vi "Call Measure.vi"(0 "Measurement Client Wrapper in":refnum<class "Measurement Client Wrapper.lvclass">, 5 "Config Data":T2(array[cluster]), 7 "Expected Output Format":T2(array[cluster]), 9 "ConfigurationParametersMessagetype":string, 11 "error in (no error)":errorcluster) -> (4 "Measurement Client Wrapper out":refnum<class "Measurement Client Wrapper.lvclass">, 6 "Output Data":T2(array[cluster]), 15 "error out":errorcluster)   [LabVIEW 2020, in "Measurement Client Wrapper.lvclass"]
uses:
  Measurement Client Wrapper.lvclass
  Typedefs/Measurement DataType.ctl
  Measurement Client Wrapper.lvclass/Measurement Client Wrapper.ctl
  <vilib>/gRPC/LabVIEW gRPC Library/Server API/typeDefs/Message Element Type.ctl
  02400f1b-8973-4b95-8741-fbceca04c3fe.vi
  5b726686-77e5-40ef-be8d-2074d1d57e99.vi
  95b28ee5-f8e2-4b34-8d76-37da75901063.vi
  00fa3f71-b6c4-4477-9b91-f6e537aa3dd8.vi
  5907dd95-356c-493c-a4fb-246df12ff7d4.vi
  c2266674-1d71-4ea2-b566-157aa4afc0f2.vi
  1a1b2748-f9f2-4ce1-9d96-6eb652a988f1.vi
  d543a457-6964-494b-8b0b-6a35ff49fad2.vi
  99282071-cc29-4e12-a9c1-055a10bff9dc.vi
  d266cb79-5d95-441f-85b0-bd6ef5cfb0df.vi
  03ab3711-fcfd-4277-a820-7570fda2cb30.vi
  0c734c18-9f5b-4fb1-9d32-7552b2f84713.vi
  e636cc20-c55c-4ee7-9f06-d3ba27ad9f12.vi
  7d8d1cdd-67f0-488f-acda-45a393ef5429.vi
  dec23bc4-0ee6-41f8-bde8-6d2a7e7bdfda.vi
  0367a431-a951-4815-abe7-6dcef05fe4c8.vi
  10f836c9-6199-4ce1-a626-5162e79beb86.vi
  96ee5240-0b84-4974-8ad0-9b306673ed4a.vi
  d29134f8-404b-4b6f-a3af-5734ff761ebd.vi
  181fb914-151b-4e06-975b-9dc9e5afafa5.vi
  588d01ac-b7df-4f6b-8274-d762d09c065e.vi
  c5a5b341-584b-41e8-87a1-35fc57d4ddfd.vi
  f3bca736-9bdf-40e5-ab0d-7db104ab277d.vi
  6802ca25-6fd7-49a0-8882-e0466137b412.vi
  c7c6e655-8529-4469-afec-6f432153ed64.vi
  520864e9-ee10-48de-be12-7897d471816d.vi
  46e9815d-b5c5-41d7-ada4-ba252c25d075.vi
  bc126205-1da4-432e-a22b-db4c055c1324.vi
  e14ad0fc-2d1f-4c15-8e45-af447a0faebc.vi
  407f5415-5085-4ddd-a591-6d04ba5119ca.vi
  af61a386-2c35-4d4b-91aa-3cbffd5e8033.vi
  97c6c522-6e58-44d8-a6ef-9522c331f38e.vi
  <vilib>/gRPC/LabVIEW gRPC Library/Server API/Server/Get Server DLL Path.vi
  Measurement_lv_client/Measurement_lv_client Class/Measurement_lv_client.lvclass
  <vilib>/gRPC/LabVIEW gRPC Library/gprc-lvsupport-release.lvlib
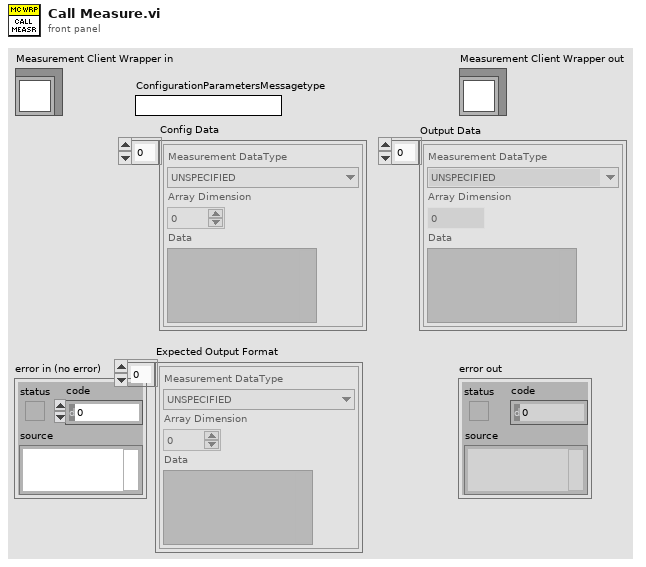
[diagram p1: front panel]
types:
  T1 = typedef "Measurement Client Wrapper.lvclass/Measurement DataType.ctl" = enum16{"UNSPECIFIED", "BOOL", "DOUBLE", "FLOAT", "INT32", "INT64", "STRING", "UINT32", "UINT64"}
  T2 = cluster{"Measurement DataType":T1, "Array Dimension":i32, "Data":variant}[]
  T3 = typedef "gprc-lvsupport-release.lvlib/Message Element Type.ctl" = enum32{"Int32Value", "FloatValue", "DoubleValue", "BoolValue", "StringValue", "MessageValue", "Int64Value", "UInt32Value", "UInt64Value", "EnumValue", "Bytes", "Fixed64", "Fixed32", "SFixed64", "SFixed32", "SInt64", "SInt32"}
  T4 = typedef "gprc-lvsupport-release.lvlib/grpcId.ctl" = u64
  T5 = typedef "Measurement_lv_client.lvlib/Measurement_lv_client.lvclass/Measurement_v1_MeasureResponse_Data.ctl" = cluster{"outputs":T6, "Error":T7}
  T6 = typedef "Measurement_lv_client.lvlib/Measurement_lv_client.lvclass/google_protobuf_Any_Data.ctl" = cluster{"type_url":string, "value":u8[]}
  T7 = typedef "Measurement_lv_client.lvlib/Measurement_lv_client.lvclass/Measurement_v1_ErrorInformation_Data.ctl" = cluster{"iserror":bool, "errorcode":i32, "errordetails":string}
  T8 = cluster{"Measurement DataType":T1, "Array Dimension":i32, "Data":variant}
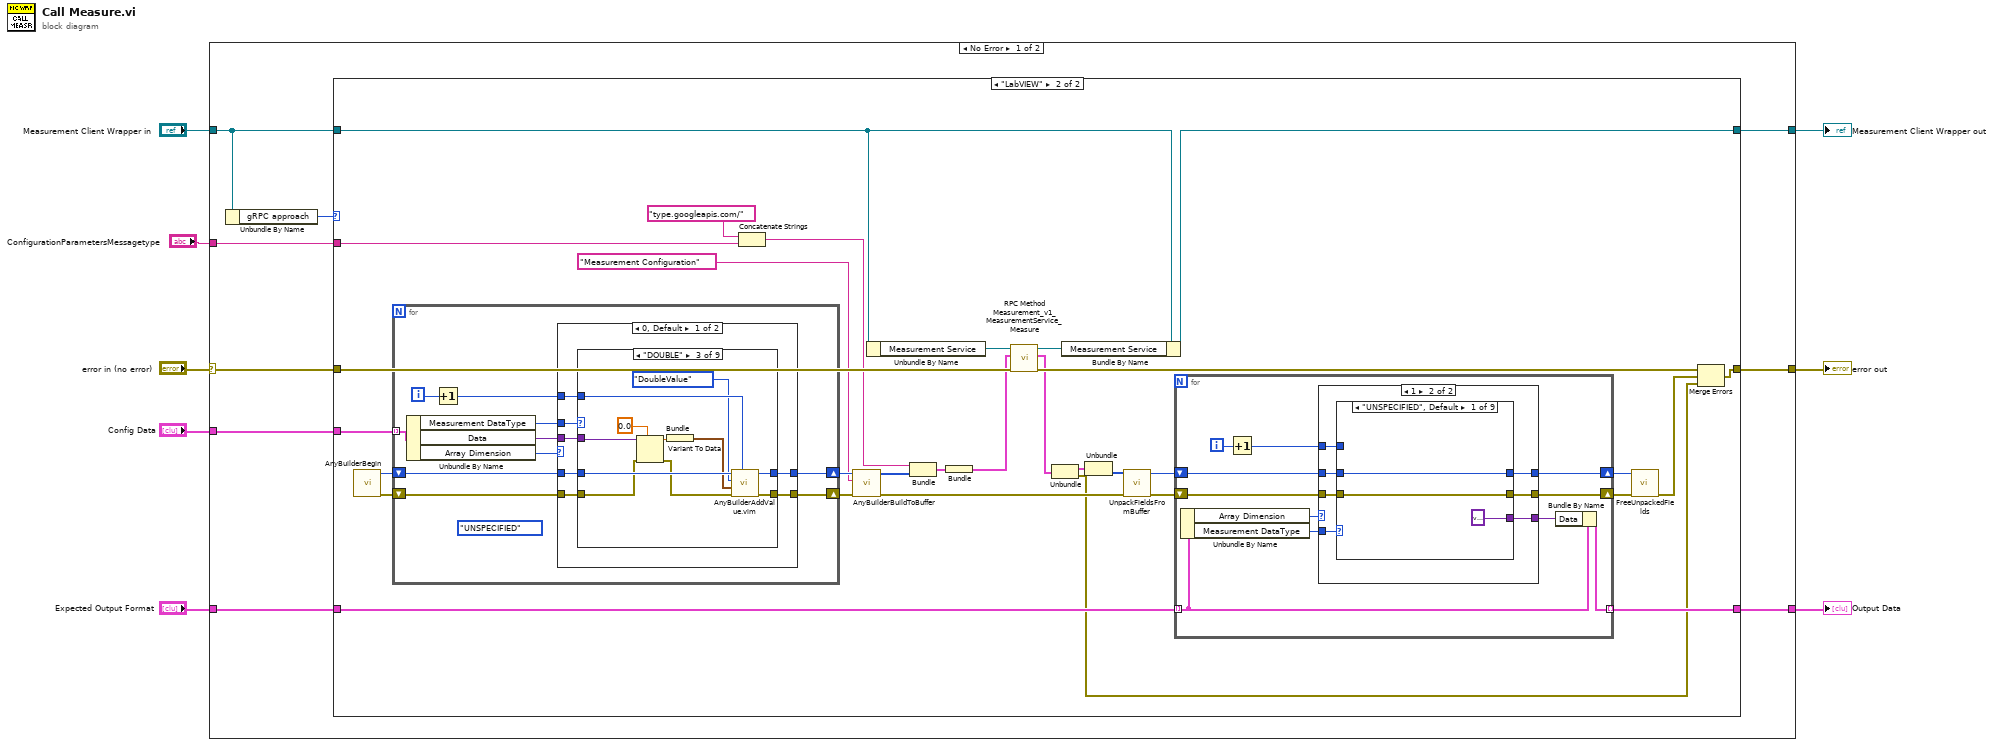
[diagram p0: block diagram]
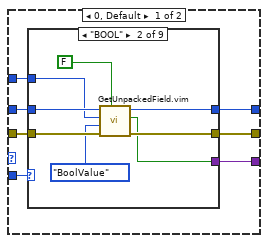
[diagram p3: hidden frame]
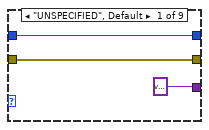
[diagram p4: hidden frame]
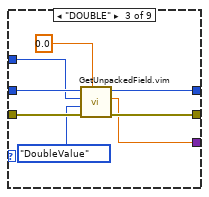
[diagram p5: hidden frame]
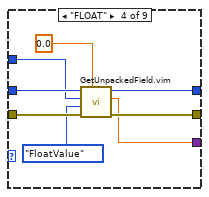
[diagram p6: hidden frame]
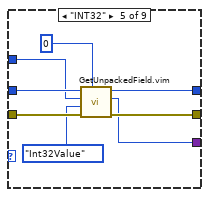
[diagram p7: hidden frame]
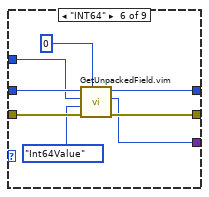
[diagram p8: hidden frame]
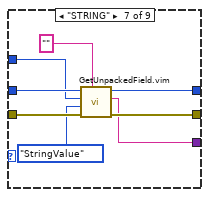
[diagram p9: hidden frame]
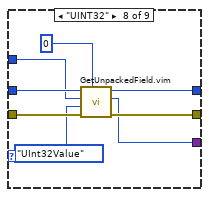
[diagram p10: hidden frame]
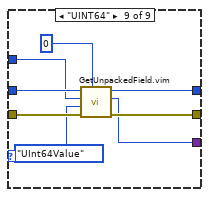
[diagram p11: hidden frame]
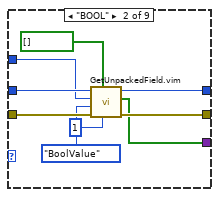
[diagram p12: hidden frame]
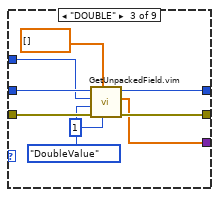
[diagram p13: hidden frame]
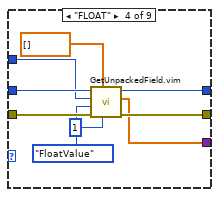
[diagram p14: hidden frame]
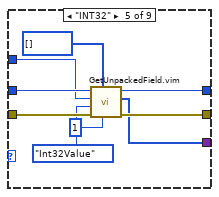
[diagram p15: hidden frame]
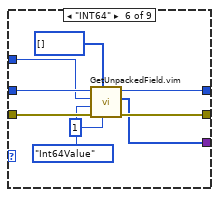
[diagram p16: hidden frame]
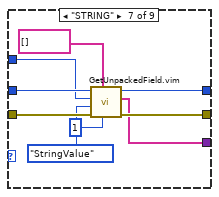
[diagram p17: hidden frame]
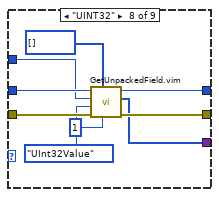
[diagram p18: hidden frame]
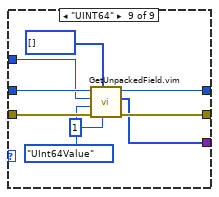
[diagram p19: hidden frame]
diagram:
  n1 = case shown="No Error" "error in (no error)" {
    selector: "error in (no error)" -> [w17 w432]
    tunnel: [w16 w432] -> w7
    tunnel: [w15 w431] -> w5
    tunnel: "Measurement Client Wrapper in" -> [w14 w431]
    tunnel: "Config Data" -> [w12 _]
    tunnel: "Expected Output Format" -> [w11 _]
    tunnel: [w10 _] -> w2
    tunnel: "ConfigurationParametersMessagetype" -> [w9 _]
    frame No Error {
      n2 = Unbundle By Name(w14) -> ("gRPC approach"=w13:enum16{".NET", "LabVIEW"})
      n3 = case shown="\"LabVIEW\"" w13 {
        tunnel: w17 -> [w20 w50]
        tunnel: [w20 w37] -> w16
        tunnel: [w19 w47] -> w15
        tunnel: w14 -> [w19 w48]
        tunnel: w12 -> [_ w45]
        tunnel: w11 -> [w18 w32]
        tunnel: [w18 w29] -> w10
        tunnel: w9 -> [_ w21]
        frame ".NET", Default {
        }
        frame "LabVIEW" {
          n4 = call <vilib>:"AnyBuilderBegin.vi"() -> ("error out"=w44:errorcluster, "Builder Ref Out"=w43:T4)  [unwired: 9 in]
          n5 = for {
            tunnel: w45 -> [w228] mode=indexing
            shift-right: [w222] -> w41
            shift-left: w44 -> [w221]
            shift-right: [w223] -> w42
            shift-left: w43 -> [w224]
            i -> [w227]
            (unwired) Measurement_DataType."UNSPECIFIED" ("Measurement DataType")
            n6 = Unbundle By Name(w228) -> ("Measurement DataType"=w226:T1, "Data"=w225:variant, "Array Dimension"=w219:i32)
            n7 = Increment(x=w227) -> (x+1=w220:i32)
            n8 = case shown="0, Default" w219 {
              tunnel: w226 -> [w235 w332]
              tunnel: w225 -> [w234 w331]
              tunnel: w224 -> [w233 w330]
              tunnel: [w232 w329] -> w223
              tunnel: [w231 w328] -> w222
              tunnel: w221 -> [w230 w327]
              tunnel: w220 -> [w229 w326]
              frame 0, Default {
                n9 = case shown="\"DOUBLE\"" w235 {
                  tunnel: w234 -> [_ w243 w254 w265 w276 w287 w298 w309 w320]
                  tunnel: w233 -> [w237 w248 w259 w270 w281 w292 w303 w314 w325]
                  tunnel: [w237 w247 w258 w269 w280 w291 w302 w313 w324] -> w232
                  tunnel: [w236 w246 w257 w268 w279 w290 w301 w312 w323] -> w231
                  tunnel: w230 -> [w236 w241 w253 w264 w275 w286 w297 w308 w319]
                  tunnel: w229 -> [_ w245 w256 w267 w278 w289 w300 w311 w322]
                  frame "UNSPECIFIED", Default {
                  }
                  frame "BOOL" {
                    n10 = Variant To Data(error in=w241, type=TRUE, Variant=w243) -> (data=w239:bool, error out=w240:errorcluster)
                    n11 = Bundle(w239) -> (w238:cluster{bool})  [unwired: 1 in]
                    n12 = call "AnyBuilderAddValue.vim"("protobufId"=w245, "error in (no error)"=w240, "Value"=w238, "MessageElementType"=Message_Element_Type."BoolValue", "gRPCid in"=w248) -> ("error out"=w246:errorcluster, "gRPCid"=w247:u64)  [unwired: 5 in]
                  }
                  frame "DOUBLE" {
                    n13 = Variant To Data(error in=w253, type=0.0, Variant=w254) -> (data=w249:dbl, error out=w252:errorcluster)
                    n14 = Bundle(w249) -> (w251:cluster{dbl})  [unwired: 1 in]
                    n15 = call "AnyBuilderAddValue.vim"("protobufId"=w256, "error in (no error)"=w252, "Value"=w251, "MessageElementType"=Message_Element_Type."DoubleValue", "gRPCid in"=w259) -> ("error out"=w257:errorcluster, "gRPCid"=w258:u64)  [unwired: 5 in]
                  }
                  frame "FLOAT" {
                    n16 = Variant To Data(error in=w264, type=sgl 0.0, Variant=w265) -> (data=w261:sgl, error out=w263:errorcluster)
                    n17 = Bundle(w261) -> (w260:cluster{sgl})  [unwired: 1 in]
                    n18 = call "AnyBuilderAddValue.vim"("protobufId"=w267, "error in (no error)"=w263, "Value"=w260, "MessageElementType"=Message_Element_Type."FloatValue", "gRPCid in"=w270) -> ("error out"=w268:errorcluster, "gRPCid"=w269:u64)  [unwired: 5 in]
                  }
                  frame "INT32" {
                    n19 = Variant To Data(error in=w275, type=0, Variant=w276) -> (data=w272:i32, error out=w274:errorcluster)
                    n20 = Bundle(w272) -> (w271:cluster{i32})  [unwired: 1 in]
                    n21 = call "AnyBuilderAddValue.vim"("protobufId"=w278, "error in (no error)"=w274, "Value"=w271, "MessageElementType"=Message_Element_Type."Int32Value", "gRPCid in"=w281) -> ("error out"=w279:errorcluster, "gRPCid"=w280:u64)  [unwired: 5 in]
                  }
                  frame "INT64" {
                    n22 = Variant To Data(error in=w286, type=i64 0, Variant=w287) -> (data=w283:i64, error out=w285:errorcluster)
                    n23 = Bundle(w283) -> (w282:cluster{i64})  [unwired: 1 in]
                    n24 = call "AnyBuilderAddValue.vim"("protobufId"=w289, "error in (no error)"=w285, "Value"=w282, "MessageElementType"=Message_Element_Type."Int64Value", "gRPCid in"=w292) -> ("error out"=w290:errorcluster, "gRPCid"=w291:u64)  [unwired: 5 in]
                  }
                  frame "STRING" {
                    n25 = Variant To Data(error in=w297, type="", Variant=w298) -> (data=w294:string, error out=w296:errorcluster)
                    n26 = Bundle(w294) -> (w293:cluster{string})  [unwired: 1 in]
                    n27 = call "AnyBuilderAddValue.vim"("protobufId"=w300, "error in (no error)"=w296, "Value"=w293, "MessageElementType"=Message_Element_Type."StringValue", "gRPCid in"=w303) -> ("error out"=w301:errorcluster, "gRPCid"=w302:u64)  [unwired: 5 in]
                  }
                  frame "UINT32" {
                    n28 = Variant To Data(error in=w308, type=u32 0, Variant=w309) -> (data=w305:u32, error out=w307:errorcluster)
                    n29 = Bundle(w305) -> (w304:cluster{u32})  [unwired: 1 in]
                    n30 = call "AnyBuilderAddValue.vim"("protobufId"=w311, "error in (no error)"=w307, "Value"=w304, "MessageElementType"=Message_Element_Type."UInt32Value", "gRPCid in"=w314) -> ("error out"=w312:errorcluster, "gRPCid"=w313:u64)  [unwired: 5 in]
                  }
                  frame "UINT64" {
                    n31 = Variant To Data(error in=w319, type=u64 0, Variant=w320) -> (data=w316:u64, error out=w318:errorcluster)
                    n32 = Bundle(w316) -> (w315:cluster{u64})  [unwired: 1 in]
                    n33 = call "AnyBuilderAddValue.vim"("protobufId"=w322, "error in (no error)"=w318, "Value"=w315, "MessageElementType"=Message_Element_Type."UInt64Value", "gRPCid in"=w325) -> ("error out"=w323:errorcluster, "gRPCid"=w324:u64)  [unwired: 5 in]
                  }
                }
              }
              frame 1 {
                n34 = case shown="\"BOOL\"" w332 {
                  tunnel: w331 -> [_ w341 w353 w365 w377 w389 w401 w413 w425]
                  tunnel: w330 -> [w334 w346 w358 w370 w382 w394 w406 w418 w430]
                  tunnel: [w334 w345 w357 w369 w381 w393 w405 w417 w429] -> w329
                  tunnel: [w333 w344 w356 w368 w380 w392 w404 w416 w428] -> w328
                  tunnel: w327 -> [w333 w340 w352 w364 w376 w388 w400 w412 w424]
                  tunnel: w326 -> [_ w343 w355 w367 w379 w391 w403 w415 w427]
                  frame "UNSPECIFIED", Default {
                  }
                  frame "BOOL" {
                    n35 = Variant To Data(error in=w340, type=bool[] [], Variant=w341) -> (data=w338:bool[], error out=w339:errorcluster)
                    n36 = Bundle(w338) -> (w337:cluster{bool[]})  [unwired: 1 in]
                    n37 = call "AnyBuilderAddValue.vim"("isRepeated"=1, "protobufId"=w343, "error in (no error)"=w339, "Value"=w337, "MessageElementType"=Message_Element_Type."BoolValue", "gRPCid in"=w346) -> ("error out"=w344:errorcluster, "gRPCid"=w345:u64)  [unwired: 4 in]
                  }
                  frame "DOUBLE" {
                    n38 = Variant To Data(error in=w352, type=dbl[] [], Variant=w353) -> (data=w349:dbl[], error out=w351:errorcluster)
                    n39 = Bundle(w349) -> (w350:cluster{dbl[]})  [unwired: 1 in]
                    n40 = call "AnyBuilderAddValue.vim"("isRepeated"=1, "protobufId"=w355, "error in (no error)"=w351, "Value"=w350, "MessageElementType"=Message_Element_Type."DoubleValue", "gRPCid in"=w358) -> ("error out"=w356:errorcluster, "gRPCid"=w357:u64)  [unwired: 4 in]
                  }
                  frame "FLOAT" {
                    n41 = Variant To Data(error in=w364, type=sgl[] [], Variant=w365) -> (data=w362:sgl[], error out=w363:errorcluster)
                    n42 = Bundle(w362) -> (w361:cluster{sgl[]})  [unwired: 1 in]
                    n43 = call "AnyBuilderAddValue.vim"("isRepeated"=1, "protobufId"=w367, "error in (no error)"=w363, "Value"=w361, "MessageElementType"=Message_Element_Type."FloatValue", "gRPCid in"=w370) -> ("error out"=w368:errorcluster, "gRPCid"=w369:u64)  [unwired: 4 in]
                  }
                  frame "INT32" {
                    n44 = Variant To Data(error in=w376, type=i32[] [], Variant=w377) -> (data=w374:i32[], error out=w375:errorcluster)
                    n45 = Bundle(w374) -> (w373:cluster{i32[]})  [unwired: 1 in]
                    n46 = call "AnyBuilderAddValue.vim"("isRepeated"=1, "protobufId"=w379, "error in (no error)"=w375, "Value"=w373, "MessageElementType"=Message_Element_Type."Int32Value", "gRPCid in"=w382) -> ("error out"=w380:errorcluster, "gRPCid"=w381:u64)  [unwired: 4 in]
                  }
                  frame "INT64" {
                    n47 = Variant To Data(error in=w388, type=i64[] [], Variant=w389) -> (data=w386:i64[], error out=w387:errorcluster)
                    n48 = Bundle(w386) -> (w385:cluster{i64[]})  [unwired: 1 in]
                    n49 = call "AnyBuilderAddValue.vim"("isRepeated"=1, "protobufId"=w391, "error in (no error)"=w387, "Value"=w385, "MessageElementType"=Message_Element_Type."Int64Value", "gRPCid in"=w394) -> ("error out"=w392:errorcluster, "gRPCid"=w393:u64)  [unwired: 4 in]
                  }
                  frame "STRING" {
                    n50 = Variant To Data(error in=w400, type=string[] [], Variant=w401) -> (data=w398:string[], error out=w399:errorcluster)
                    n51 = Bundle(w398) -> (w397:cluster{string[]})  [unwired: 1 in]
                    n52 = call "AnyBuilderAddValue.vim"("isRepeated"=1, "protobufId"=w403, "error in (no error)"=w399, "Value"=w397, "MessageElementType"=Message_Element_Type."StringValue", "gRPCid in"=w406) -> ("error out"=w404:errorcluster, "gRPCid"=w405:u64)  [unwired: 4 in]
                  }
                  frame "UINT32" {
                    n53 = Variant To Data(error in=w412, type=u32[] [], Variant=w413) -> (data=w410:u32[], error out=w411:errorcluster)
                    n54 = Bundle(w410) -> (w409:cluster{u32[]})  [unwired: 1 in]
                    n55 = call "AnyBuilderAddValue.vim"("isRepeated"=1, "protobufId"=w415, "error in (no error)"=w411, "Value"=w409, "MessageElementType"=Message_Element_Type."UInt32Value", "gRPCid in"=w418) -> ("error out"=w416:errorcluster, "gRPCid"=w417:u64)  [unwired: 4 in]
                  }
                  frame "UINT64" {
                    n56 = Variant To Data(error in=w424, type=u64[] [], Variant=w425) -> (data=w422:u64[], error out=w423:errorcluster)
                    n57 = Bundle(w422) -> (w421:cluster{u64[]})  [unwired: 1 in]
                    n58 = call "AnyBuilderAddValue.vim"("isRepeated"=1, "protobufId"=w427, "error in (no error)"=w423, "Value"=w421, "MessageElementType"=Message_Element_Type."UInt64Value", "gRPCid in"=w430) -> ("error out"=w428:errorcluster, "gRPCid"=w429:u64)  [unwired: 4 in]
                  }
                }
              }
            }
          }
          n59 = Concatenate Strings("type.googleapis.com/", w21) -> (w22:string)
          n60 = call <vilib>:"AnyBuilderBuildToBuffer.vi"("error in (no error)"=w41, "Message Type"="Measurement Configuration", "Builder Ref"=w42) -> ("error out"=w33:errorcluster, "Buffer"=w40:u8[])  [unwired: 7 in]
          n61 = Unbundle By Name(w48) -> ("Measurement Service"=w51:refnum<class "Measurement_lv_client.lvclass">)
          n62 = Bundle(w22, "Buffer"=w40) -> (w39:cluster{string, "Buffer":u8[]})  [unwired: 1 in]
          n63 = Bundle(w39) -> (w38:cluster{cluster{string, "Buffer":u8[]}})  [unwired: 1 in]
          n64 = call "RPC Method Measurement_v1_MeasurementService_Measure.vi"("error in (no error)"=w50, "Request Data"=w38, "gRPC Client in"=w51) -> ("error out"=w49:errorcluster, "Response Data"=w36:T5, "gRPC Client out"=w46:refnum<class "Measurement_lv_client.lvclass">)  [unwired: 6 in]
          n65 = Unbundle(w36) -> ("outputs"=w35:T6, "Error"=w28:T7)
          n66 = Bundle By Name(cluster=w48, "Measurement Service"=w46) -> (w47:refnum<class "Measurement Client Wrapper.lvclass">)
          n67 = Unbundle(w35) -> ("value"=w34:u8[])  [unwired: 1 out]
          n68 = call <vilib>:"UnpackFieldsFromBuffer.vi"("error in (no error)"=w33, "Buffer"=w34) -> ("error out"=w30:errorcluster, "Fields Ref Out"=w31:T4)  [unwired: 8 in]
          n69 = for {
            tunnel: w32 -> [w55] mode=indexing
            shift-right: [w60] -> w27
            shift-left: w31 -> [w61]
            shift-right: [w58] -> w26
            shift-left: w30 -> [w59]
            tunnel: [w53] -> w29 mode=indexing
            i -> [w57]
            n70 = Unbundle By Name(w55) -> ("Array Dimension"=w52:i32, "Measurement DataType"=w62:T1)
            n71 = Increment(x=w57) -> (x+1=w56:i32)
            n72 = case shown="1" w52 {
              tunnel: w62 -> [w69 w143]
              tunnel: w61 -> [w68 w142]
              tunnel: [w67 w141] -> w60
              tunnel: w59 -> [w66 w140]
              tunnel: [w65 w139] -> w58
              tunnel: w56 -> [w64 w138]
              tunnel: [w63 w137] -> w54
              frame 0, Default {
                n73 = case shown="\"BOOL\"" w69 {
                  tunnel: w68 -> [w72 w80 w88 w96 w104 w112 w120 w128 w136]
                  tunnel: [w72 w78 w86 w94 w102 w110 w118 w126 w134] -> w67
                  tunnel: w66 -> [w71 w79 w87 w95 w103 w111 w119 w127 w135]
                  tunnel: [w71 w77 w85 w93 w101 w109 w117 w125 w133] -> w65
                  tunnel: w64 -> [_ w75 w83 w91 w99 w107 w115 w123 w131]
                  tunnel: [variant w73 w81 w89 w97 w105 w113 w121 w129] -> w63
                  frame "UNSPECIFIED", Default {
                  }
                  frame "BOOL" {
                    n74 = call "GetUnpackedField.vim"("Value"=FALSE, "error in (no error)"=w79, "MessageElementType"=Message_Element_Type."BoolValue", "protobufId"=w75, "gRPCid in"=w80) -> ("error out"=w77:errorcluster, "value"=w73:bool, "gRPCid"=w78:u64)  [unwired: 4 in]
                  }
                  frame "DOUBLE" {
                    n75 = call "GetUnpackedField.vim"("Value"=0.0, "error in (no error)"=w87, "MessageElementType"=Message_Element_Type."DoubleValue", "protobufId"=w83, "gRPCid in"=w88) -> ("error out"=w85:errorcluster, "value"=w81:dbl, "gRPCid"=w86:u64)  [unwired: 4 in]
                  }
                  frame "FLOAT" {
                    n76 = call "GetUnpackedField.vim"("Value"=sgl 0.0, "error in (no error)"=w95, "MessageElementType"=Message_Element_Type."FloatValue", "protobufId"=w91, "gRPCid in"=w96) -> ("error out"=w93:errorcluster, "value"=w89:sgl, "gRPCid"=w94:u64)  [unwired: 4 in]
                  }
                  frame "INT32" {
                    n77 = call "GetUnpackedField.vim"("Value"=0, "error in (no error)"=w103, "MessageElementType"=Message_Element_Type."Int32Value", "protobufId"=w99, "gRPCid in"=w104) -> ("error out"=w101:errorcluster, "value"=w97:i32, "gRPCid"=w102:u64)  [unwired: 4 in]
                  }
                  frame "INT64" {
                    n78 = call "GetUnpackedField.vim"("Value"=i64 0, "error in (no error)"=w111, "MessageElementType"=Message_Element_Type."Int64Value", "protobufId"=w107, "gRPCid in"=w112) -> ("error out"=w109:errorcluster, "value"=w105:i64, "gRPCid"=w110:u64)  [unwired: 4 in]
                  }
                  frame "STRING" {
                    n79 = call "GetUnpackedField.vim"("Value"="", "error in (no error)"=w119, "MessageElementType"=Message_Element_Type."StringValue", "protobufId"=w115, "gRPCid in"=w120) -> ("error out"=w117:errorcluster, "value"=w113:string, "gRPCid"=w118:u64)  [unwired: 4 in]
                  }
                  frame "UINT32" {
                    n80 = call "GetUnpackedField.vim"("Value"=u32 0, "error in (no error)"=w127, "MessageElementType"=Message_Element_Type."UInt32Value", "protobufId"=w123, "gRPCid in"=w128) -> ("error out"=w125:errorcluster, "value"=w121:u32, "gRPCid"=w126:u64)  [unwired: 4 in]
                  }
                  frame "UINT64" {
                    n81 = call "GetUnpackedField.vim"("Value"=u64 0, "error in (no error)"=w135, "MessageElementType"=Message_Element_Type."UInt64Value", "protobufId"=w131, "gRPCid in"=w136) -> ("error out"=w133:errorcluster, "value"=w129:u64, "gRPCid"=w134:u64)  [unwired: 4 in]
                  }
                }
              }
              frame 1 {
                n82 = case shown="\"UNSPECIFIED\", Default" w143 {
                  tunnel: w142 -> [w146 w155 w164 w173 w182 w191 w200 w209 w218]
                  tunnel: [w146 w153 w162 w171 w180 w189 w198 w207 w216] -> w141
                  tunnel: w140 -> [w145 w154 w163 w172 w181 w190 w199 w208 w217]
                  tunnel: [w145 w152 w161 w170 w179 w188 w197 w206 w215] -> w139
                  tunnel: w138 -> [_ w151 w160 w169 w178 w187 w196 w205 w214]
                  tunnel: [variant w149 w158 w167 w176 w185 w194 w203 w212] -> w137
                  frame "UNSPECIFIED", Default {
                  }
                  frame "BOOL" {
                    n83 = call "GetUnpackedField.vim"("isRepeated"=1, "Value"=bool[] [], "error in (no error)"=w154, "MessageElementType"=Message_Element_Type."BoolValue", "protobufId"=w151, "gRPCid in"=w155) -> ("error out"=w152:errorcluster, "value"=w149:bool[], "gRPCid"=w153:u64)  [unwired: 3 in]
                  }
                  frame "DOUBLE" {
                    n84 = call "GetUnpackedField.vim"("isRepeated"=1, "Value"=dbl[] [], "error in (no error)"=w163, "MessageElementType"=Message_Element_Type."DoubleValue", "protobufId"=w160, "gRPCid in"=w164) -> ("error out"=w161:errorcluster, "value"=w158:dbl[], "gRPCid"=w162:u64)  [unwired: 3 in]
                  }
                  frame "FLOAT" {
                    n85 = call "GetUnpackedField.vim"("isRepeated"=1, "Value"=sgl[] [], "error in (no error)"=w172, "MessageElementType"=Message_Element_Type."FloatValue", "protobufId"=w169, "gRPCid in"=w173) -> ("error out"=w170:errorcluster, "value"=w167:sgl[], "gRPCid"=w171:u64)  [unwired: 3 in]
                  }
                  frame "INT32" {
                    n86 = call "GetUnpackedField.vim"("isRepeated"=1, "Value"=i32[] [], "error in (no error)"=w181, "MessageElementType"=Message_Element_Type."Int32Value", "protobufId"=w178, "gRPCid in"=w182) -> ("error out"=w179:errorcluster, "value"=w176:i32[], "gRPCid"=w180:u64)  [unwired: 3 in]
                  }
                  frame "INT64" {
                    n87 = call "GetUnpackedField.vim"("isRepeated"=1, "Value"=i64[] [], "error in (no error)"=w190, "MessageElementType"=Message_Element_Type."Int64Value", "protobufId"=w187, "gRPCid in"=w191) -> ("error out"=w188:errorcluster, "value"=w185:i64[], "gRPCid"=w189:u64)  [unwired: 3 in]
                  }
                  frame "STRING" {
                    n88 = call "GetUnpackedField.vim"("isRepeated"=1, "Value"=string[] [], "error in (no error)"=w199, "MessageElementType"=Message_Element_Type."StringValue", "protobufId"=w196, "gRPCid in"=w200) -> ("error out"=w197:errorcluster, "value"=w194:string[], "gRPCid"=w198:u64)  [unwired: 3 in]
                  }
                  frame "UINT32" {
                    n89 = call "GetUnpackedField.vim"("isRepeated"=1, "Value"=u32[] [], "error in (no error)"=w208, "MessageElementType"=Message_Element_Type."UInt32Value", "protobufId"=w205, "gRPCid in"=w209) -> ("error out"=w206:errorcluster, "value"=w203:u32[], "gRPCid"=w207:u64)  [unwired: 3 in]
                  }
                  frame "UINT64" {
                    n90 = call "GetUnpackedField.vim"("isRepeated"=1, "Value"=u64[] [], "error in (no error)"=w217, "MessageElementType"=Message_Element_Type."UInt64Value", "protobufId"=w214, "gRPCid in"=w218) -> ("error out"=w215:errorcluster, "value"=w212:u64[], "gRPCid"=w216:u64)  [unwired: 3 in]
                  }
                }
              }
            }
            n91 = Bundle By Name(cluster=w55, "Data"=w54) -> (w53:T8)
          }
          n92 = call <vilib>:"FreeUnpackedFields.vi"("error in (no error)"=w26, "Unpacked Fields ID"=w27) -> ("error out"=w25:errorcluster)  [unwired: 9 in]
          n93 = Merge Errors(w49, w25, w28) -> (w37:errorcluster)
        }
      }
    }
    frame Error {
    }
  }
  "error out" <- w7
  "Measurement Client Wrapper out" <- w5
  "Output Data" <- w2
